vi "HeaderuRayon.vi"(0 "Oper.":string, 1 "VR":string, 2 "S/N":string, 3 "UUT":string, 4 "UA":string, 5 "UUTHeader":string, 7 "Revision Param":string, 8 "Tester Software Ver":string) -> (6 "HEADER1":string)   [LabVIEW 2017]
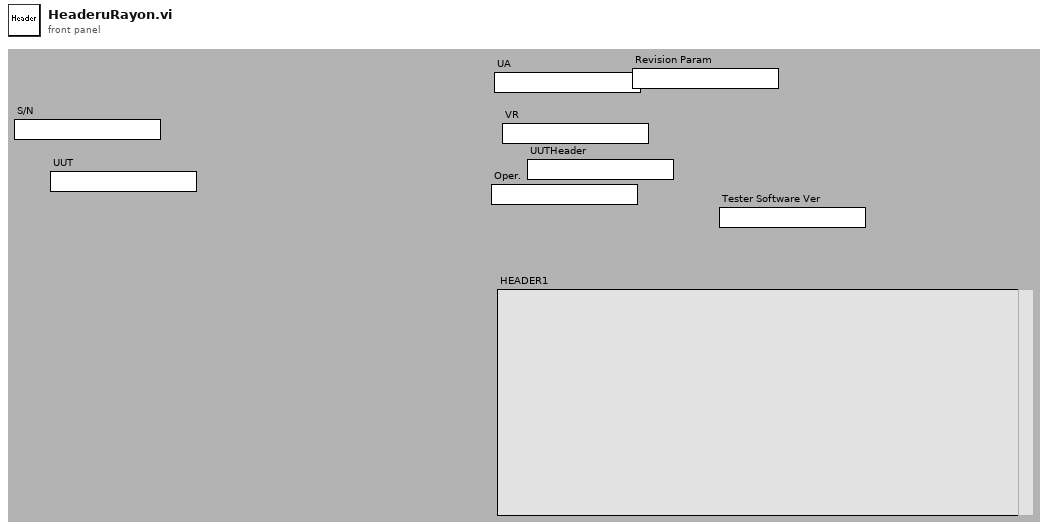
[diagram p1: front panel]
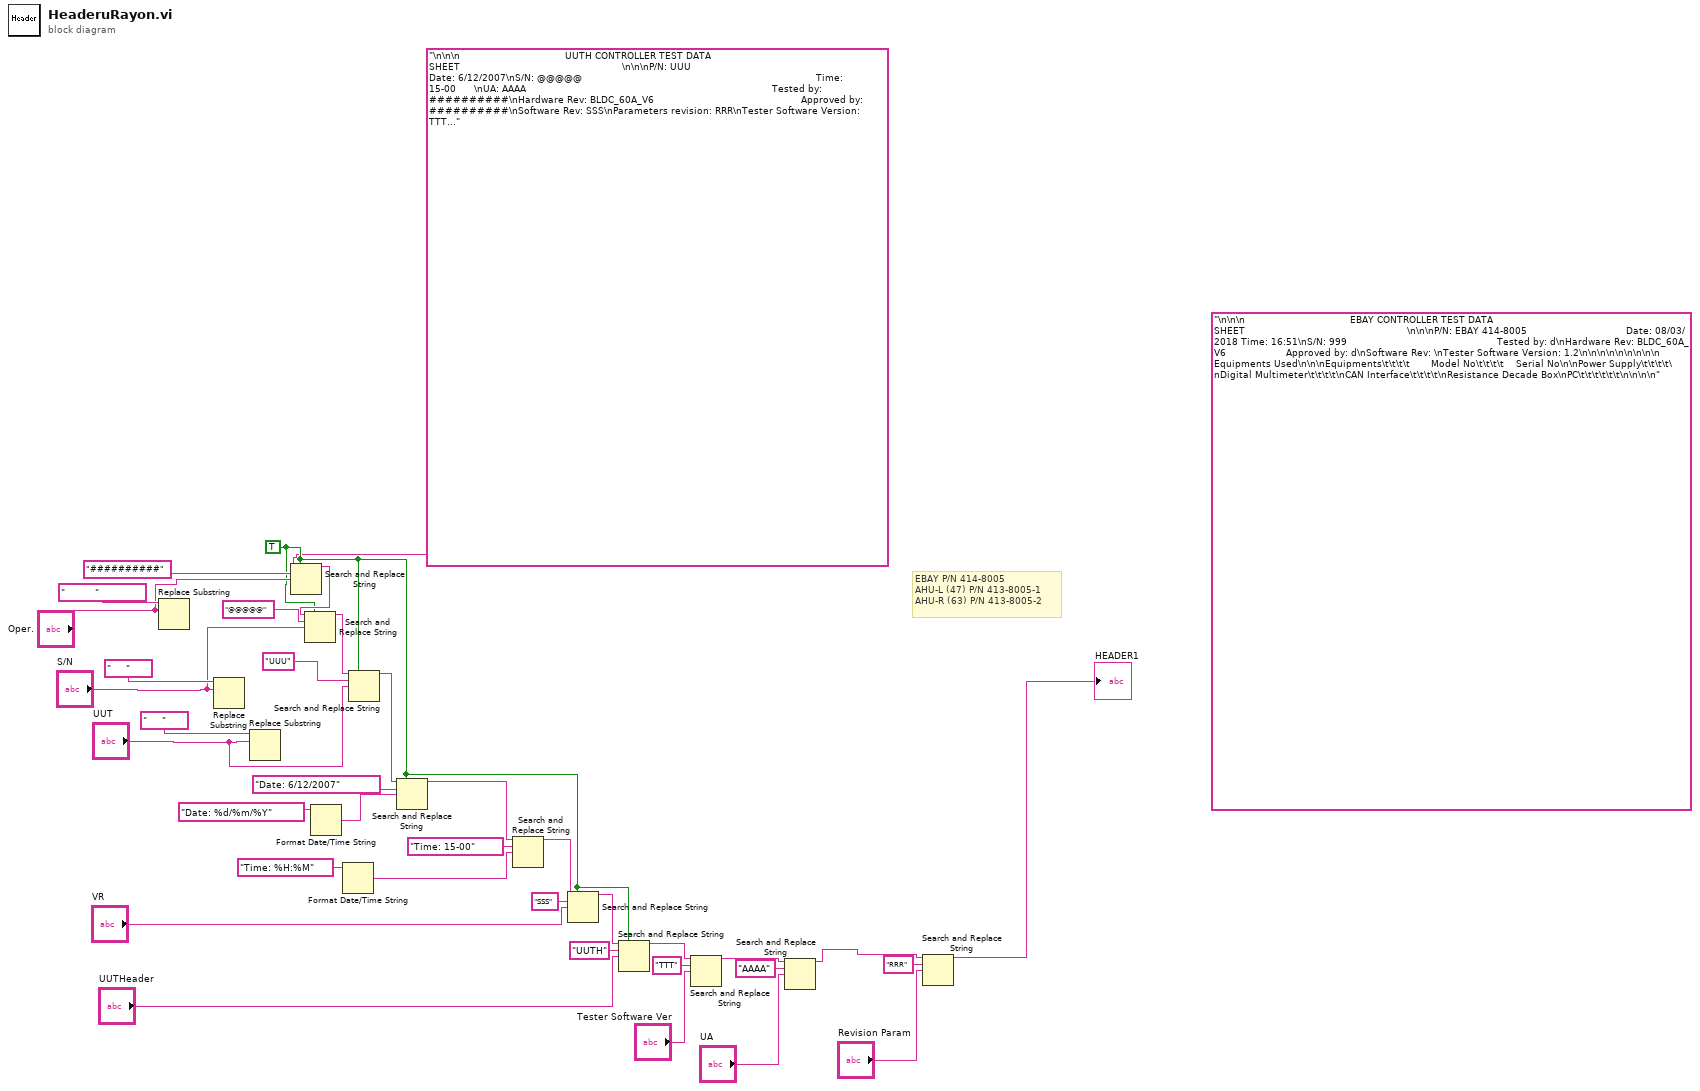
[diagram p0: block diagram]
diagram:
  (unwired) "\n\n\n                                   EBAY CONTROLLER TEST DATA SHEET                                                      \n\n\nP/N: EBAY 414-8005                                 Date: 08/03/2018 Time: 16:51\nS/N: 999                                                  Tested by: d\nHardware Rev: BLDC_60A_V6                    Approved by: d\nSoftware Rev: \nTester Software Version: 1.2\n\n\n\n\n\n\n\n\n                                                Equipments Used\n\n\nEquipments\t\t\t\t       Model No\t\t\t\t    Serial No\n\nPower Supply\t\t\t\t\nDigital Multimeter\t\t\t\t\nCAN Interface\t\t\t\t\nResistance Decade Box\nPC\t\t\t\t\t\t\n\n\n\n" ("HEADER1 2")
  w19 = TRUE ("replace all? (F)")
  # "EBAY P/N 414-8005\nAHU-L (47) P/N 413-8005-1\nAHU-R (63) P/N 413-8005-2"
  n1 = Replace Substring(4:"Oper.", 5:"          " ("source")) -> ()  [unwired: 2 in, 2 out]
  n2 = Replace Substring(4:"S/N", 5:"     " ("source")) -> ()  [unwired: 2 in, 2 out]
  n3 = Replace Substring(4:"UUT", 5:"     " ("source")) -> ()  [unwired: 2 in, 2 out]
  n4 = Search and Replace String(replace all?=w19, input string="\n\n\n                                   UUTH CONTROLLER TEST DATA SHEET                                                      \n\n\nP/N: UUU                                                               Date: 6/12/2007\nS/N: @@@@@                                                                              Time: 15-00      \nUA: AAAA                                                                                  Tested by: ##########\nHardware Rev: BLDC_60A_V6                                                 Approved by: ##########\nSoftware Rev: SSS\nParameters revision: RRR\nTester Software Version: TTT\n\n\n\n\n\n                                                Equipments Used\n\n\nEquipments\t\t\t\t       Model No\t\t\t\t    Serial No\n\nPower Supply\t\t\t\t\nDigital Multimeter\t\t\t\t\nCAN Interface\t\t\t\t\nBLDC Tester\nPC\t\t\t\t\t\t\nHeater\nRS-232 Interface\nCurrent Meter" ("result string"), search string="##########" ("source"), replace string="Oper.") -> (result string=w32:string)  [unwired: 4 in, 3 out]
  n5 = Search and Replace String(replace all?=w19, input string=w32, search string="@@@@@" ("source"), replace string="S/N") -> (result string=w27:string)  [unwired: 4 in, 3 out]
  n6 = Format Date/Time String(time format string (%c)="Date: %d/%m/%Y") -> (date/time string=w36:string)  [unwired: 2 in]
  n7 = Format Date/Time String(time format string (%c)="Time: %H:%M") -> (date/time string=w5:string)  [unwired: 2 in]
  n8 = Search and Replace String(replace all?=w19, input string=w27, search string="UUU" ("source"), replace string="UUT") -> (result string=w28:string)  [unwired: 4 in, 3 out]
  n9 = Search and Replace String(replace all?=w19, input string=w28, search string="Date: 6/12/2007" ("time format string (%c)"), replace string=w36) -> (result string=w8:string)  [unwired: 4 in, 3 out]
  n10 = Search and Replace String(input string=w8, search string="Time: 15-00", replace string=w5) -> (result string=w7:string)  [unwired: 5 in, 3 out]
  n11 = Search and Replace String(replace all?=w19, input string=w7, search string="SSS", replace string="VR") -> (result string=w20:string)  [unwired: 4 in, 3 out]
  n12 = Search and Replace String(replace all?=w19, input string=w20, search string="UUTH", replace string="UUTHeader") -> (result string=w15:string)  [unwired: 4 in, 3 out]
  n13 = Search and Replace String(input string=w15, search string="TTT", replace string="Tester Software Ver") -> (result string=w12:string)  [unwired: 5 in, 3 out]
  n14 = Search and Replace String(input string=w12, search string="AAAA", replace string="UA") -> (result string=w2:string)  [unwired: 5 in, 3 out]
  n15 = Search and Replace String(input string=w2, search string="RRR", replace string="Revision Param") -> (result string=→"HEADER1":string)  [unwired: 5 in, 3 out]
